vi "Read Temperature.vi"(8 "error in (no error)":errorcluster, 11 "ThermPID in":refnum<class "ThermPID.lvclass">) -> (0 "error out":errorcluster, 1 "Output (V)":dbl, 2 "Temperature (C)":dbl, 3 "ThermPID out":refnum<class "ThermPID.lvclass">)   [LabVIEW 2023, in "ThermPID.lvclass"]
uses:
  ThermPID.lvclass
  ThermPID.lvclass/ThermPID.ctl
  PIDController/PIDController.lvclass
  <vilib>/NI/Modbus Library/API/Master/Modbus Master.lvclass
  PIDModBus/Controls/Register Enum.ctl
  PIDModBus/PIDModbus.lvlib
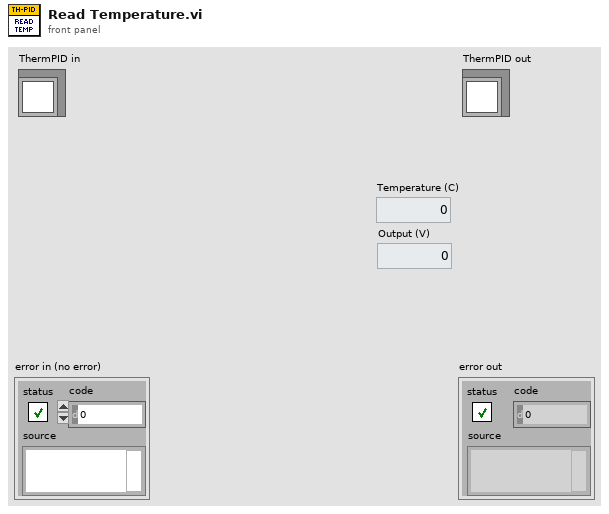
[diagram p1: front panel]
types:
  T1 = typedef "PIDModbus.lvlib/Register Enum.ctl" = u16
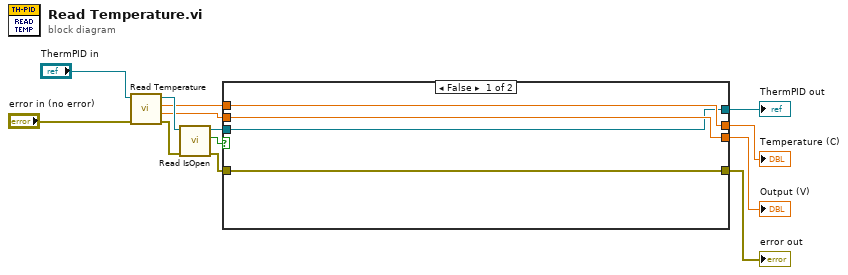
[diagram p0: block diagram]
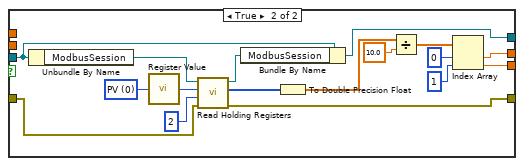
[diagram p2: hidden frame]
diagram:
  n1 = call-parent "Read Temperature.vi"("error in (no error)"="error in (no error)", "PIDController in"="ThermPID in") -> ("error out"=w6:errorcluster, "Output (V)"=w2:dbl, "Temperature (C)"=w1:dbl, "PIDController out"=w13:refnum<class "ThermPID.lvclass">)  [unwired: 6 in]
  n2 = call-dynamic "Read IsOpen.vi"("error in (no error)"=w6, "PIDController in"=w13) -> ("error out"=w5:errorcluster, "IsOpen"=w3:bool, "PIDController out"=w4:refnum<class "ThermPID.lvclass">)  [unwired: 7 in]
  n3 = case shown="False" w3 {
    tunnel: [w16 w25] -> w10
    tunnel: [w17 w24] -> w9
    tunnel: [w14 w23] -> w8
    tunnel: [w15 w22] -> w7
    tunnel: w5 -> [w14 w20]
    tunnel: w4 -> [w15 w19]
    tunnel: w2 -> [w17 _]
    tunnel: w1 -> [w16 _]
    frame False {
    }
    frame True {
      w32 = T1 0 items=["PV"=0, "SV"=5, "P1"=24, "I1"=25, "D1"=26] ("Register")
      n4 = Unbundle By Name(w19) -> ("ModbusSession"=w18:refnum<class "Modbus Master.lvclass">)
      n5 = call "Register Value.vi"("Register"=w32) -> ("RegAddr (Hex)"=w31:u16)
      n6 = call-dynamic "Read Holding Registers.vi"("error in"=w20, "number of inputs"=u16 2, "starting address"=w31, "Modbus master in"=w18) -> ("error out"=w23:errorcluster, "register values"=w34:u16[], "Modbus master out"=w21:refnum<class "Modbus Master.lvclass">)  [unwired: 5 in]
      n7 = Bundle By Name(cluster=w19, "ModbusSession"=w21) -> (w22:refnum<class "ThermPID.lvclass">)
      n8 = To Double Precision Float(number=w34) -> (double precision float=w29:dbl[])
      n9 = Divide(x=w29, y=10.0) -> (x/y=w28:dbl[])
      n10 = Index Array(array=w28, index #1=0 ("index"), index #2=1 ("index")) -> (element #1=w25:dbl, element #2=w24:dbl)
    }
  }
  "error out" <- w8
  "ThermPID out" <- w7
  "Temperature (C)" <- w10
  "Output (V)" <- w9
